vi "cursor-moveSD.vi"(1 "cluster in":T1={"Experiments groups"=[], "Kinetics"=[], "Spectrum"=[], "GRAPH EXPERIMENTAL DATA"=[], "kinetics plot names"=[], "spectra plot names"=[], "group"=0, "exp selected"=0, "# exp"=0, "error out"={"status"=FALSE, "code"=0, "source"=""}, "FromToWave"={"FromWave"=0.0, "ToWave"=0.0}, "GRAPH EXPERIMENTAL DATA ref"=refnum, "timedelays"=[0.0, 0.0, 0.0, 0.0, 0.0, 0.0, 0.0, 0.06019061100911815, 0.0521779104562645, 0.045231877429679615, 0.03921051490799832, 0.033990728811568754, 0.029465811603150715, 0.025543260876973825, 0.02214288834180205, 0.01919518054014414, 0.016639877791965713, 0.014424742312398925, 0.012504490320209958, 0.010839866306230088, 0.009396840537117498, 0.008145913389103785, 0.00706151229029317, 0.006121468943269439, 0.005306566140927374, 0.004600144911132549, 0.003987763959109073, 0.0034569044455719407, 0.00299671406541447, 0.0025977851951783253, 0.0022519625739982996, 0.00195217658646366, 0.0016922987392150965, 0.0014670163768006634, 0.0012717240756200802, 0.0011024294957352762, 0.0009556717658856477, 0.0008284507332614981, 0.0007181656316962257, 0.0006225619144775864, 0.0005396851648867825, 0.00046784114226338394, 0.0004055611468220084, 0.0003515719951773376, 0.00030476999279031153, 0.00026419837125694315, 0.00022902772919263772, 0.0001985390768670671, 0.0001721091379728629, 0.00014919760805372974, 0.00012933610911736794], "wavelengths"=[0.0, 0.0, 0.0, 0.0, 0.0, 0.0, 0.0, 0.06019061100911815, 0.0521779104562645, 0.045231877429679615, 0.03921051490799832, 0.033990728811568754, 0.029465811603150715, 0.025543260876973825, 0.02214288834180205, 0.01919518054014414, 0.016639877791965713, 0.014424742312398925, 0.012504490320209958, 0.010839866306230088, 0.009396840537117498, 0.008145913389103785, 0.00706151229029317, 0.006121468943269439, 0.005306566140927374, 0.004600144911132549, 0.003987763959109073, 0.0034569044455719407, 0.00299671406541447, 0.0025977851951783253, 0.0022519625739982996, 0.00195217658646366, 0.0016922987392150965, 0.0014670163768006634, 0.0012717240756200802, 0.0011024294957352762, 0.0009556717658856477, 0.0008284507332614981, 0.0007181656316962257, 0.0006225619144775864, 0.0005396851648867825, 0.00046784114226338394, 0.0004055611468220084, 0.0003515719951773376, 0.00030476999279031153, 0.00026419837125694315, 0.00022902772919263772, 0.0001985390768670671, 0.0001721091379728629, 0.00014919760805372974, 0.00012933610911736794], "Experiment"=refnum, "Commentaires exp"=refnum, "FromToDelay"={"FromDelay"=0.0, "ToDelay"=0.0}}, 2 "User Event in":refnum<user-event>) -> (0 "output out":T1={"Experiments groups"=[], "Kinetics"=[], "Spectrum"=[], "GRAPH EXPERIMENTAL DATA"=[], "kinetics plot names"=[], "spectra plot names"=[], "group"=0, "exp selected"=0, "# exp"=0, "error out"={"status"=FALSE, "code"=0, "source"=""}, "FromToWave"={"FromWave"=0.0, "ToWave"=0.0}, "GRAPH EXPERIMENTAL DATA ref"=refnum, "timedelays"=[0.0, 0.0, 0.0, 0.0, 0.0, 0.0, 0.0, 0.06019061100911815, 0.0521779104562645, 0.045231877429679615, 0.03921051490799832, 0.033990728811568754, 0.029465811603150715, 0.025543260876973825, 0.02214288834180205, 0.01919518054014414, 0.016639877791965713, 0.014424742312398925, 0.012504490320209958, 0.010839866306230088, 0.009396840537117498, 0.008145913389103785, 0.00706151229029317, 0.006121468943269439, 0.005306566140927374, 0.004600144911132549, 0.003987763959109073, 0.0034569044455719407, 0.00299671406541447, 0.0025977851951783253, 0.0022519625739982996, 0.00195217658646366, 0.0016922987392150965, 0.0014670163768006634, 0.0012717240756200802, 0.0011024294957352762, 0.0009556717658856477, 0.0008284507332614981, 0.0007181656316962257, 0.0006225619144775864, 0.0005396851648867825, 0.00046784114226338394, 0.0004055611468220084, 0.0003515719951773376, 0.00030476999279031153, 0.00026419837125694315, 0.00022902772919263772, 0.0001985390768670671, 0.0001721091379728629, 0.00014919760805372974, 0.00012933610911736794], "wavelengths"=[0.0, 0.0, 0.0, 0.0, 0.0, 0.0, 0.0, 0.06019061100911815, 0.0521779104562645, 0.045231877429679615, 0.03921051490799832, 0.033990728811568754, 0.029465811603150715, 0.025543260876973825, 0.02214288834180205, 0.01919518054014414, 0.016639877791965713, 0.014424742312398925, 0.012504490320209958, 0.010839866306230088, 0.009396840537117498, 0.008145913389103785, 0.00706151229029317, 0.006121468943269439, 0.005306566140927374, 0.004600144911132549, 0.003987763959109073, 0.0034569044455719407, 0.00299671406541447, 0.0025977851951783253, 0.0022519625739982996, 0.00195217658646366, 0.0016922987392150965, 0.0014670163768006634, 0.0012717240756200802, 0.0011024294957352762, 0.0009556717658856477, 0.0008284507332614981, 0.0007181656316962257, 0.0006225619144775864, 0.0005396851648867825, 0.00046784114226338394, 0.0004055611468220084, 0.0003515719951773376, 0.00030476999279031153, 0.00026419837125694315, 0.00022902772919263772, 0.0001985390768670671, 0.0001721091379728629, 0.00014919760805372974, 0.00012933610911736794], "Experiment"=refnum, "Commentaires exp"=refnum, "FromToDelay"={"FromDelay"=0.0, "ToDelay"=0.0}})   [LabVIEW 2015]
uses:
  controls/control-cluster.ctl
  Classes/Experiments_group.lvclass
types:
  T1 = typedef "control-cluster.ctl" = cluster{"Experiments groups":refnum<class "Experiments_group.lvclass">[], "Kinetics":cluster{"timedelay":dbl[], dbl[]}[], "Spectrum":cluster{"Unités abscisse":dbl[], dbl[]}[], "GRAPH EXPERIMENTAL DATA":dbl[][], "kinetics plot names":string[], "spectra plot names":string[], "group":i32, "exp selected":i32, "# exp":i32, "error out":errorcluster, "FromToWave":cluster{"FromWave":dbl, "ToWave":dbl}, "GRAPH EXPERIMENTAL DATA ref":refnum<vi>, "timedelays":dbl[], "wavelengths":dbl[], "Experiment":refnum<vi>, "Commentaires exp":refnum<vi>, "FromToDelay":cluster{"FromDelay":dbl, "ToDelay":dbl}}
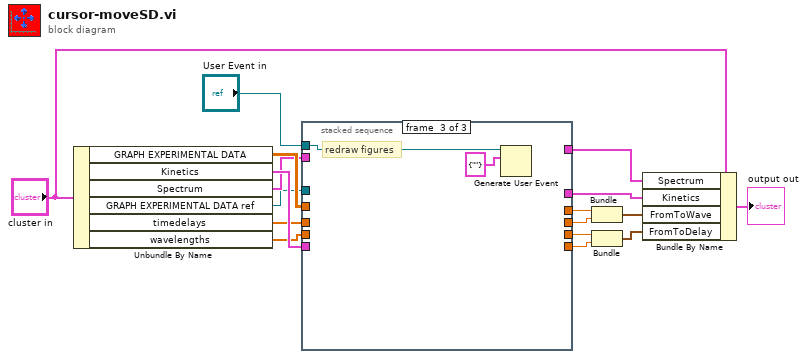
[diagram p0: block diagram]
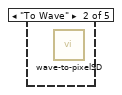
[diagram p4: hidden frame]
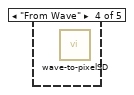
[diagram p6: hidden frame]
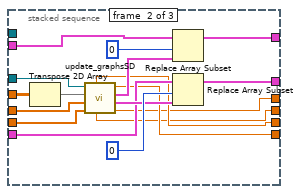
[diagram p8: hidden frame]
diagram:
  n1 = Unbundle By Name("cluster in") -> ("GRAPH EXPERIMENTAL DATA"=w16:dbl[][], "Kinetics"=w13:cluster{"timedelay":dbl[], dbl[]}[], "Spectrum"=w12:cluster{"Unités abscisse":dbl[], dbl[]}[], "GRAPH EXPERIMENTAL DATA ref"=w3:refnum<vi>, "timedelays"=w2:dbl[], "wavelengths"=w1:dbl[])
  n2 = stacked-sequence {
    tunnel: [_ w31 _] -> w14
    tunnel: [_ w36 _] -> w15
    tunnel: "User Event in" -> [_ _ w39]
    tunnel: w16 -> [_ w30 _]
    tunnel: w13 -> [_ w29 _]
    tunnel: w12 -> [_ w28 _]
    tunnel: [_ w27 _] -> w9
    tunnel: [_ w26 _] -> w8
    tunnel: [_ w25 _] -> w6
    tunnel: [_ w24 _] -> w5
    tunnel: w3 -> [_ w23 _]
    tunnel: w2 -> [_ w22 _]
    tunnel: w1 -> [_ w21 _]
    frame #0 {
      n3 = disable-structure shown="Disabled" {
        disable-tunnel: _ -> [w18 _]
        frame Disabled {
          n4 = case shown="\"GRAPH EXPERIMENTAL DATA\", Default" w18 {
            frame "To Time" {
            }
            frame "To Wave" {
              n5 = call "wave-to-pixelSD.vi"() -> ("Wave"=w19:dbl)  [unwired: 1 out]
            }
            frame "From Time" {
            }
            frame "From Wave" {
              n6 = call "wave-to-pixelSD.vi"() -> ("Wave"=w20:dbl)  [unwired: 1 out]
            }
            frame "GRAPH EXPERIMENTAL DATA", Default {
            }
          }
        }
        frame Enabled {
        }
      }
    }
    frame #1 {
      n7 = Transpose 2D Array(2D array=w30) -> (transposed array=w37:dbl[][])
      n8 = call "update_graphsSD.vi"("wavelengths"=w21, "timedelays"=w22, "data"=w37, "IntensityGraph in"=w23) -> ("From wave"=w25:dbl, "Kinetics"=w34:cluster{"timedelay":dbl[], dbl[]}[], "Spectrum"=w32:cluster{"Unités abscisse":dbl[], dbl[]}[], "To time"=w27:dbl, "To wave"=w24:dbl, "From  time"=w26:dbl)
      n9 = Replace Array Subset(array=w28, new element=w32, index=0) -> (w31:cluster{"Unités abscisse":dbl[], dbl[]}[])
      n10 = Replace Array Subset(array=w29, new element=w34, index=0) -> (w36:cluster{"timedelay":dbl[], dbl[]}[])
    }
    frame #2 {
      # "redraw figures"
      n11 = Generate User Event(user event=w39, event data cluster=cluster{"what to redraw":string} {"what to redraw"=""} ("event data")) -> ()  [unwired: 2 in, 2 out]
    }
  }
  n12 = Bundle("From wave"=w6, "To wave"=w5) -> (w4:cluster{"From wave":dbl, "To wave":dbl})  [unwired: 1 in]
  n13 = Bundle("From  time"=w8, "To time"=w9) -> (w7:cluster{"From  time":dbl, "To time":dbl})  [unwired: 1 in]
  n14 = Bundle By Name(cluster="cluster in", "Spectrum"=w14, "Kinetics"=w15, "FromToWave"=w4, "FromToDelay"=w7) -> (→"output out":T1)
